vi "SRS830_Read2Channel.vi"(8 "error in (no error)":errorcluster, 11 "Lock in\nGPIB Address":i16) -> (0 "error out":errorcluster, 2 "Ch_OUTP3":dbl, 3 "Ch_OUTR1":dbl)   [LabVIEW 2014]
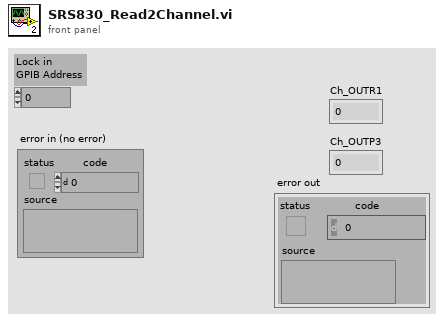
[diagram p1: front panel]
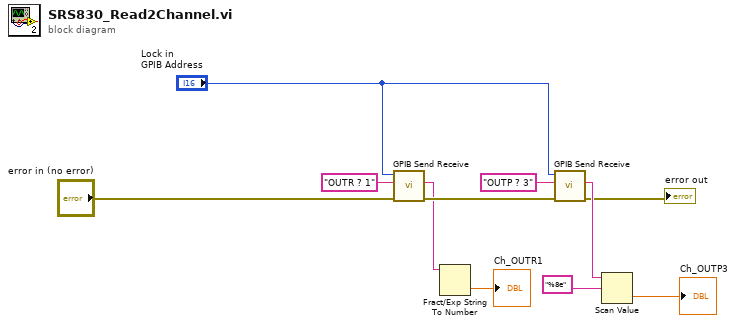
[diagram p0: block diagram]
diagram:
  n1 = call "GPIB Send Receive.vi"("error in (no error)"="error in (no error)", "data string in"="OUTR ? 1", "GPIB Adress"="Lock in\nGPIB Address") -> ("error out"=w8:errorcluster, "data string out"=w7:string)  [unwired: 6 in, 1 out]
  n2 = Fract/Exp String To Number(string=w7) -> (number=→"Ch_OUTR1":dbl)  [unwired: 3 in, 1 out]
  n3 = call "GPIB Send Receive.vi"("error in (no error)"=w8, "data string in"="OUTP ? 3", "GPIB Adress"="Lock in\nGPIB Address") -> ("error out"=→"error out":errorcluster, "data string out"=w6:string)  [unwired: 6 in, 1 out]
  n4 = Scan Value(string=w6, format string="%8e") -> (value=→"Ch_OUTP3":dbl)  [unwired: 1 in, 1 out]
